vi "Desktop Main.vi"() -> ()   [LabVIEW 2017]
doc: "Demonstrates how to use User Datagram Protocol (UDP) to send data to the myRIO target."
panel:
  in  "cupData":cluster{"X":dbl, "Y":dbl, "h_ratio":dbl}
  out "Image Out":T1(plugin-control)
  out "error out":errorcluster
  in  "Target IP Address":string="172.22.11.2"
  # "Overview: Demonstrates how to use User Datagram Protocol (UDP) to send data to the myRIO target.\nInstructions:\n1. Verify if the value of Target IP Address is correct. If not, specify the correct value.\n2. Run this VI.\n3. Open RT Main.vi and follow its front panel instructions.\n4. Change the value of LED on this VI and observe the value of LED Status on RT Main.vi.\n5. Click Stop to stop this VI."
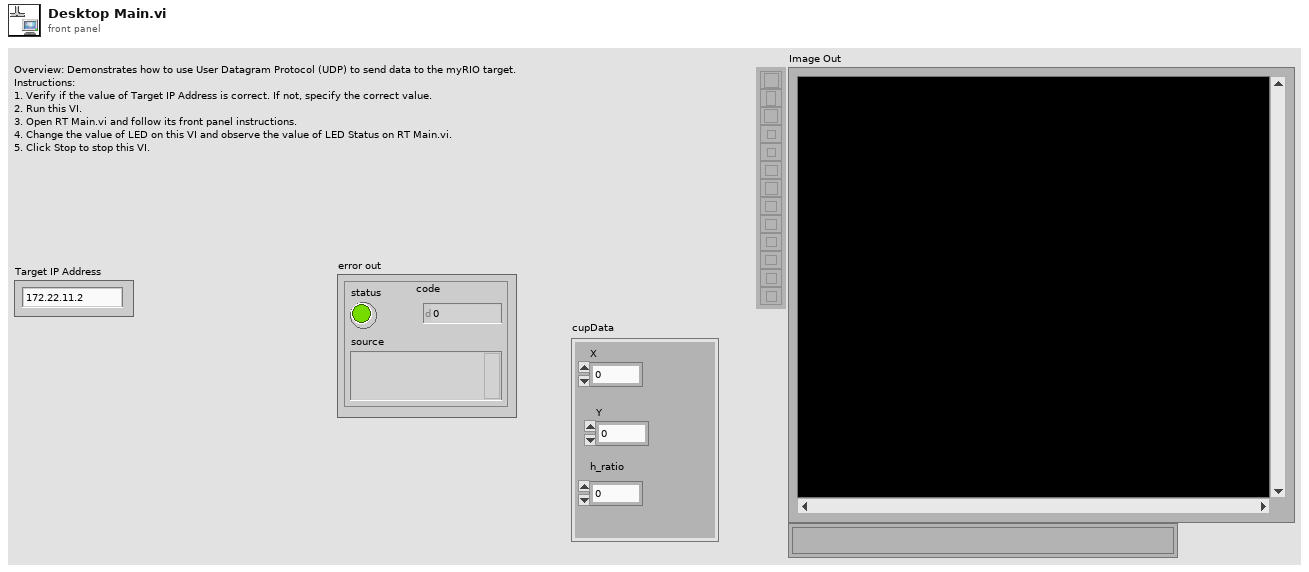
[diagram p1: front panel]
types:
  T1 = typedef "IMAQ Image.ctl" = refnum<image>
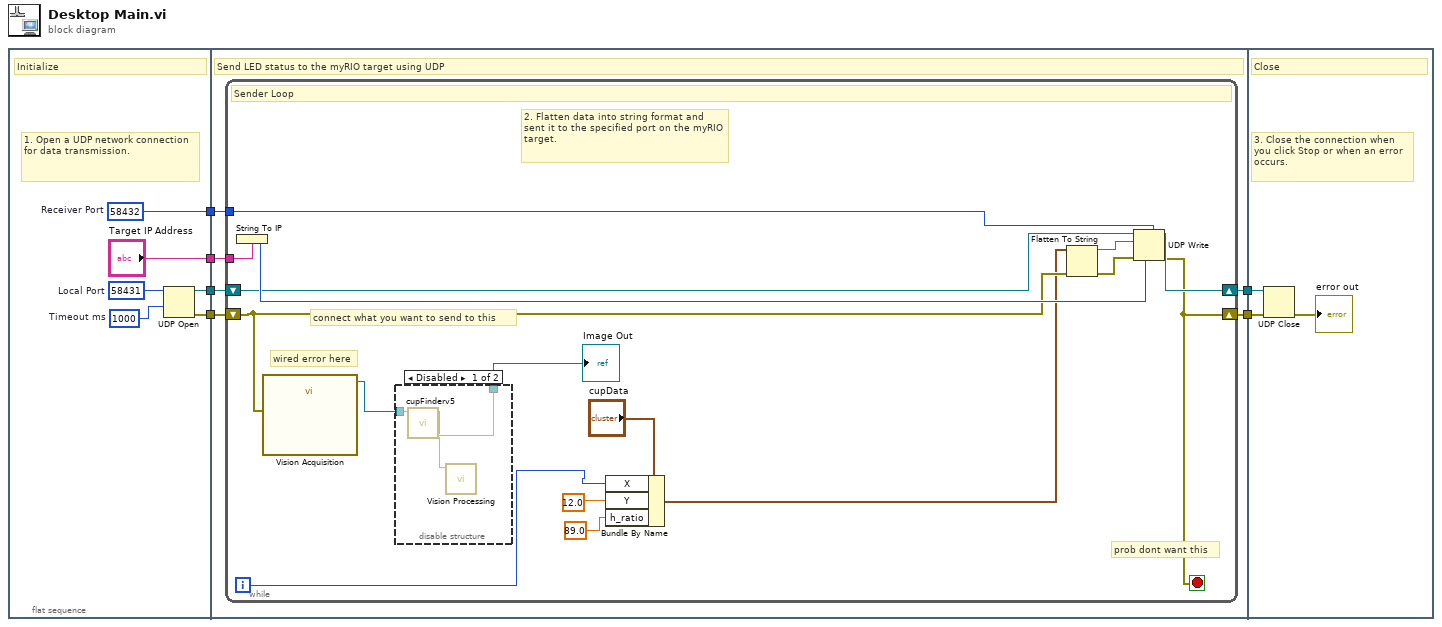
[diagram p0: block diagram]
diagram:
  n1 = flat-sequence {
    tunnel: [w11] -> w4
    tunnel: [w10] -> w3
    tunnel: ["Target IP Address"] -> w2
    tunnel: [w8] -> w1
    tunnel: [w18] -> w6
    tunnel: [w17] -> w5
    tunnel: w4 -> [w16]
    tunnel: w3 -> [w15]
    tunnel: w2 -> [w14]
    tunnel: w1 -> [w13]
    tunnel: w6 -> [w38]
    tunnel: w5 -> [w39]
    frame #0 {
      w7 = 1000  # Timeout ms
      w8 = u16 58432  # Receiver Port
      w12 = u16 58431  # Local Port
      # "1. Open a UDP network connection for data transmission."
      # "Initialize"
      n2 = UDP Open(9:w7, 11:w12) -> (port=w11:refnum<k16>, 0:w10:errorcluster)  [unwired: 3 in, 1 out]
    }
    frame #1 {
      # "Send LED status to the myRIO target using UDP"
      n3 = while {
        shift-right: [w20] -> w18
        shift-left: w15 -> [w27]
        shift-right: [w28] -> w17
        shift-left: w16 -> [w30]
        tunnel: w14 -> [w29]
        tunnel: w13 -> [w31]
        i -> [w19]
        stop <- w20 stop-if-true
        # "prob dont want this"
        # "wired error here"
        # "connect what you want to send to this"
        # "2. Flatten data into string format and\nsent it to the specified port on the myRIO target."
        # "Sender Loop"
        n4 = String To IP(1:w29) -> (0:w34:u32)
        n5 = call "Vision Acquisition"("error in"=w27) -> ("Image Out"=w25:T1)  [unwired: 23 in, 3 out]
        n6 = disable-structure shown="Disabled" {
          disable-tunnel: [w36 _] -> w26
          disable-tunnel: w25 -> [w35 _]
          frame Disabled {
            n7 = call "cupFinderv5.vi"("image\n in"=w35) -> ("WORK FOR GODS SAKE 2"=w36:T1)  [unwired: 5 in, 5 out]
            n8 = call "Vision Processing.vi"("Image In"=w35) -> ()  [unwired: 10 in, 1 out]
          }
          frame Enabled {
          }
        }
        "Image Out" <- w26
        n9 = Bundle By Name(cluster="cupData", "X"=w19, "Y"=12.0 ("Height Ratio"), "h_ratio"=89.0 ("Height Ratio")) -> (w23:cluster{"X":dbl, "Y":dbl, "h_ratio":dbl})
        n10 = Flatten To String(anything=w23, error in (no error)=w27) -> (data string=w33:string, error out=w32:errorcluster)  [unwired: 2 in, 1 out]
        n11 = UDP Write(address=w34, port or service name=w31, connection ID=w30, data in=w33, 8:w32) -> (error out=w20:errorcluster, 3:w28:refnum<k16>)  [unwired: 1 in]
      }
    }
    frame #2 {
      # "3. Close the connection when you click Stop or when an error occurs."
      # "Close"
      n12 = UDP Close(connection ID=w39, 8:w38) -> (error out=→"error out":errorcluster)  [unwired: 1 out]
    }
  }
